vi "Tree Add items.vi"(10 "Items Ct":i32, 11 "TreeControl in":refnum<vi>) -> (3 "TreeControl Out":refnum<vi>)   [LabVIEW 2023]
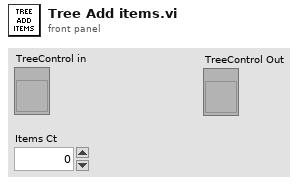
[diagram p1: front panel]
types:
  T1 = cluster{"Left Cell String":string, "Child Text":string[], "Child Tag":string, "Item Indent":i32, "Child Only?":bool, "Glyph Index":i32}
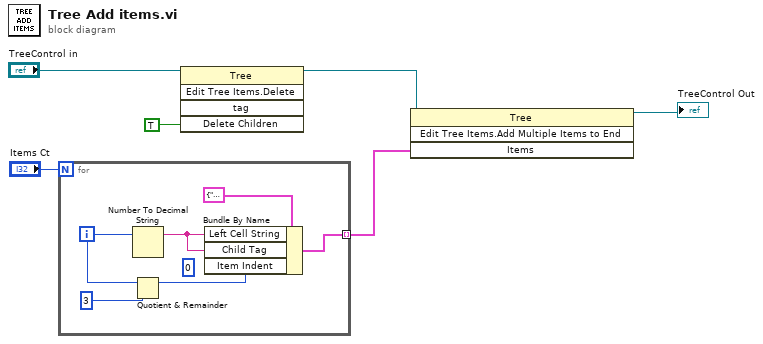
[diagram p0: block diagram]
diagram:
  n1 = for {
    N: "Items Ct" -> [_]
    tunnel: [w11] -> w6 mode=indexing
    i -> [w10]
    (unwired) 0 ("Item Indent")
    n2 = Number To Decimal String(number=w10) -> (decimal integer string=w8:string)  [unwired: 1 in]
    n3 = Quotient & Remainder(x=w10, y=3) -> (x-y*floor(x/y)=w7:i32)  [unwired: 1 out]
    n4 = Bundle By Name(cluster=T1 {"Left Cell String"="", "Child Text"=[], "Child Tag"="", "Item Indent"=0, "Child Only?"=FALSE, "Glyph Index"=0} ("Item"), "Left Cell String"=w8, "Child Tag"=w8, "Item Indent"=w7) -> (w11:T1)
  }
  n5 = invoke class="Tree" method="Edit Tree Items.Delete"(reference="TreeControl in", "Delete Children"=TRUE) -> (reference out=w1:refnum<vi>)  [unwired: 3 in, 4 out]
  n6 = invoke class="Tree" method="Edit Tree Items.Add Multiple Items to End"(reference=w1, "Items"=w6) -> (reference out=→"TreeControl Out":refnum<vi>)  [unwired: 2 in, 3 out]
